vi "Cannon Get and use.vi"(1 "Move":dbl, 2 "InTake Max":bool, 3 "Fire":bool) -> (0 "Cannon Info":T1)   [LabVIEW 2013]
uses:
  Kick Global.vi
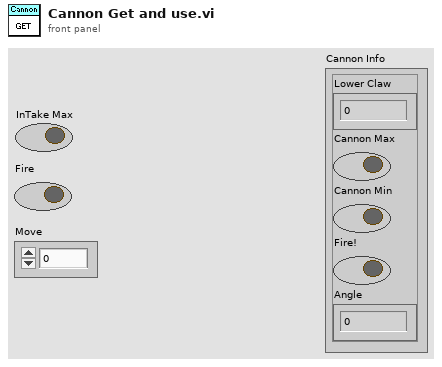
[diagram p1: front panel]
types:
  T1 = cluster{"Lower Claw":dbl, "Cannon Max":bool, "Cannon Min":bool, "Fire!":bool, "Angle":dbl}
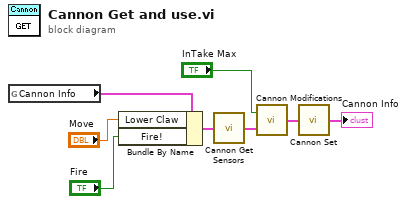
[diagram p0: block diagram]
diagram:
  n1 = global read "Kick Global.vi" "Cannon Info"() -> (w8:T1)
  n2 = Bundle By Name(cluster=w8, "Lower Claw"="Move", "Fire!"="Fire") -> (w3:T1)
  n3 = call "Cannon Get Sensors.vi"("Cannon Info"=w3) -> ("Cannon Info"=w5:T1)
  n4 = call "Cannon Modifications.vi"("Cannon Info"=w5, "InTake Max"="InTake Max") -> ("Cannon Info"=w4:T1)
  n5 = call "Cannon Set.vi"("Cannon Info"=w4) -> ("Cannon Info"=→"Cannon Info":T1)
